vi "KMC PC Main.vi"() -> ()   [LabVIEW 2014]
uses:
  <vilib>/Utility/inputDevices.llb/keyboardAcquire.vi
panel:
  out "Manual Speed":dbl
  out "Manual Rudder":dbl
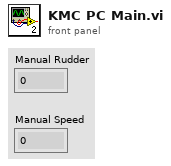
[diagram p1: front panel]
types:
  T1 = enum16{"0", "1", "2", "3", "4", "5", "6", "7", "8", "9", "A", "B", "C", "D", "E", "F", "G", "H", "I", "J", "K", "L", "M", "N", "O", "P", "Q", "R", "S", "T", "U", "V", "W", "X", "Y", "Z", "F1", "F2", "F3", "F4", "F5", "F6", "F7", "F8", "F9", "F10", "F11", "F12", "F13", "F14", "F15", "ADD", "BACK", "BACKSLASH", "CAPITAL", "COMMA", "DECIMAL", "DELETE", "DIVIDE", "DOWN", "END", "EQUALS", "ESCAPE", "GRAVE (`)", "HOME", "INSERT", "LBRACKET", "LCONTROL", "LEFT", "L ALT", "LSHIFT", "LWIN", "MINUS", "MULTIPLY", "NEXT", "NUMLOCK", "NUMPAD_0", "NUMPAD_1", "NUMPAD_2", "NUMPAD_3", "NUMPAD_4", "NUMPAD_5", "NUMPAD_6", "NUMPAD_7", "NUMPAD_8", "NUMPAD_9", "PAUSE", "PERIOD", "PRIOR (PG UP)", "RBRACKET", "RCONTROL", "RETURN", "RIGHT", "R ALT", "RSHIFT", "RWIN", "SCROLL", "SEMICOLON", "SLASH", "SPACE", "SUBTRACT", "TAB", "UP", "ENTER (num pad)", "' (quote)"}[]
  T2 = enum16{"0", "1", "2", "3", "4", "5", "6", "7", "8", "9", "A", "B", "C", "D", "E", "F", "G", "H", "I", "J", "K", "L", "M", "N", "O", "P", "Q", "R", "S", "T", "U", "V", "W", "X", "Y", "Z", "F1", "F2", "F3", "F4", "F5", "F6", "F7", "F8", "F9", "F10", "F11", "F12", "F13", "F14", "F15", "ADD", "BACK", "BACKSLASH", "CAPITAL", "COMMA", "DECIMAL", "DELETE", "DIVIDE", "DOWN", "END", "EQUALS", "ESCAPE", "GRAVE (`)", "HOME", "INSERT", "LBRACKET", "LCONTROL", "LEFT", "L ALT", "LSHIFT", "LWIN", "MINUS", "MULTIPLY", "NEXT", "NUMLOCK", "NUMPAD_0", "NUMPAD_1", "NUMPAD_2", "NUMPAD_3", "NUMPAD_4", "NUMPAD_5", "NUMPAD_6", "NUMPAD_7", "NUMPAD_8", "NUMPAD_9", "PAUSE", "PERIOD", "PRIOR (PG UP)", "RBRACKET", "RCONTROL", "RETURN", "RIGHT", "R ALT", "RSHIFT", "RWIN", "SCROLL", "SEMICOLON", "SLASH", "SPACE", "SUBTRACT", "TAB", "UP", "ENTER (num pad)", "' (quote)"}
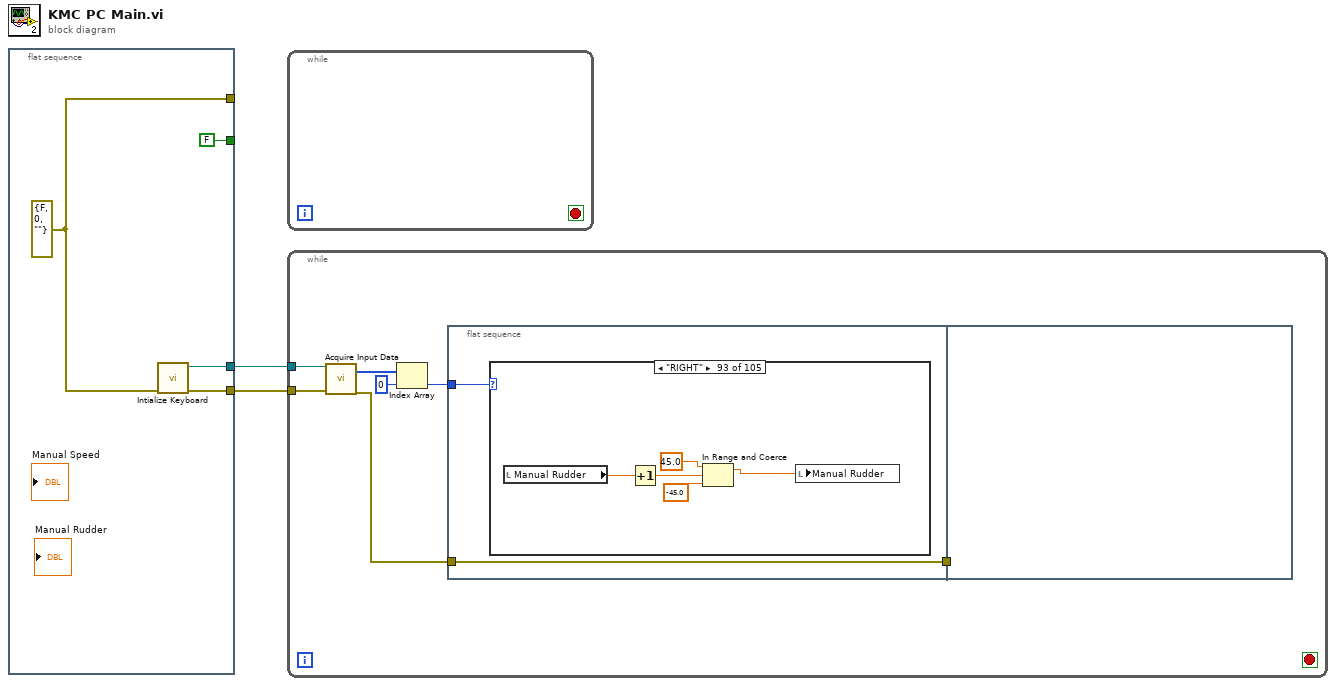
[diagram p0: block diagram]
diagram:
  n1 = flat-sequence {
    tunnel: [w6] -> _
    tunnel: [w5] -> w2
    tunnel: [w4] -> w1
    tunnel: [FALSE] -> _
    frame #0 {
      w6 = errorcluster {"status"=FALSE, "code"=0, "source"=""} ("error constant")
      n2 = call <vilib>:"Intialize Keyboard.vi"("error in (no error)"=w6) -> ("error out"=w5:errorcluster, "device ID"=w4:refnum<k1>)  [unwired: 9 in]
    }
  }
  n3 = while {
    stop <- _ stop-if-true
  }
  n4 = while {
    tunnel: w2 -> [w13]
    tunnel: w1 -> [w12]
    stop <- _ stop-if-true
    n5 = call-poly <vilib>:"Acquire Input Data.vi"("device ID"=w12, "error in (no error)"=w13) -> ("keys pressed"=w11:T1, "error out"=w7:errorcluster)  [unwired: 15 in, 1 out]
    n6 = Index Array(array=w11, index=0) -> (element=w9:T2)
    n7 = flat-sequence {
      tunnel: w9 -> [w15]
      tunnel: [w14] -> w8
      tunnel: w7 -> [w14]
      tunnel: w8 -> [_]
      frame #0 {
        n8 = case shown="\"RIGHT\"" w15 {
          frame "0", Default {
          }
          frame "1" {
          }
          frame "2" {
          }
          frame "3" {
          }
          frame "4" {
          }
          frame "5" {
          }
          frame "6" {
          }
          frame "7" {
          }
          frame "8" {
          }
          frame "9" {
          }
          frame "A" {
          }
          frame "B" {
          }
          frame "C" {
          }
          frame "D" {
          }
          frame "E" {
          }
          frame "F" {
          }
          frame "G" {
          }
          frame "H" {
          }
          frame "I" {
          }
          frame "J" {
          }
          frame "K" {
          }
          frame "L" {
          }
          frame "M" {
          }
          frame "N" {
          }
          frame "O" {
          }
          frame "P" {
          }
          frame "Q" {
          }
          frame "R" {
          }
          frame "S" {
          }
          frame "T" {
          }
          frame "U" {
          }
          frame "V" {
          }
          frame "W" {
          }
          frame "X" {
          }
          frame "Y" {
          }
          frame "Z" {
          }
          frame "F1" {
          }
          frame "F2" {
          }
          frame "F3" {
          }
          frame "F4" {
          }
          frame "F5" {
          }
          frame "F6" {
          }
          frame "F7" {
          }
          frame "F8" {
          }
          frame "F9" {
          }
          frame "F10" {
          }
          frame "F11" {
          }
          frame "F12" {
          }
          frame "F13" {
          }
          frame "F14" {
          }
          frame "F15" {
          }
          frame "ADD" {
          }
          frame "BACK" {
          }
          frame "BACKSLASH" {
          }
          frame "CAPITAL" {
          }
          frame "COMMA" {
          }
          frame "DECIMAL" {
          }
          frame "DELETE" {
          }
          frame "DIVIDE" {
          }
          frame "DOWN" {
          }
          frame "END" {
          }
          frame "EQUALS" {
          }
          frame "ESCAPE" {
          }
          frame "GRAVE (`)" {
          }
          frame "HOME" {
          }
          frame "INSERT" {
          }
          frame "LBRACKET" {
          }
          frame "LCONTROL" {
          }
          frame "LEFT" {
          }
          frame "L ALT" {
          }
          frame "LSHIFT" {
          }
          frame "LWIN" {
          }
          frame "MINUS" {
          }
          frame "MULTIPLY" {
          }
          frame "NEXT" {
          }
          frame "NUMLOCK" {
          }
          frame "NUMPAD_0" {
          }
          frame "NUMPAD_1" {
          }
          frame "NUMPAD_2" {
          }
          frame "NUMPAD_3" {
          }
          frame "NUMPAD_4" {
          }
          frame "NUMPAD_5" {
          }
          frame "NUMPAD_6" {
          }
          frame "NUMPAD_7" {
          }
          frame "NUMPAD_8" {
          }
          frame "NUMPAD_9" {
          }
          frame "PAUSE" {
          }
          frame "PERIOD" {
          }
          frame "PRIOR (PG UP)" {
          }
          frame "RBRACKET" {
          }
          frame "RCONTROL" {
          }
          frame "RETURN" {
          }
          frame "RIGHT" {
            n9 = local read "Manual Rudder"() -> (w19:dbl)
            n10 = Increment(x=w19) -> (x+1=w16:dbl)
            n11 = In Range and Coerce(upper limit=45.0, x=w16, lower limit=-45.0) -> (coerced(x)=w20:dbl)  [unwired: 1 out]
            n12 = local write "Manual Rudder"(w20) -> ()
          }
          frame "R ALT" {
          }
          frame "RSHIFT" {
          }
          frame "RWIN" {
          }
          frame "SCROLL" {
          }
          frame "SEMICOLON" {
          }
          frame "SLASH" {
          }
          frame "SPACE" {
          }
          frame "SUBTRACT" {
          }
          frame "TAB" {
          }
          frame "UP" {
          }
          frame "ENTER (num pad)" {
          }
          frame "' (quote)" {
          }
        }
      }
      frame #1 {
      }
    }
  }
